vi "Get Write Mode.vi"(8 "error in (no error)":errorcluster, 11 "Item Ref in":T2 format="%.0x") -> (0 "error out":errorcluster, 2 "Write Mode":T1, 3 "Item Ref out":T2 format="%.0x")   [LabVIEW 2020, in "Modbus Master System Explorer.lvlib"]
uses:
  Modbus Master System Explorer.lvlib
  <vilib>/NI VeriStand/Custom Device API/Custom Device Item Ref.ctl
  Shared/Write Mode.ctl
  Shared/Constants.vi
  <vilib>/NI VeriStand/Custom Device API/Get Item Property (U16).vi
  Shared/Modbus Master Shared.lvlib
  <vilib>/NI VeriStand/Custom Device API/Custom Device API.lvlib
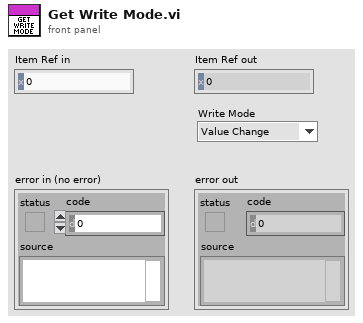
[diagram p1: front panel]
types:
  T1 = typedef "Modbus Master Shared.lvlib/Write Mode.ctl" = enum16{"Value Change", "Interval"}
  T2 = typedef "Custom Device API.lvlib/Custom Device Item Ref.ctl" = u64
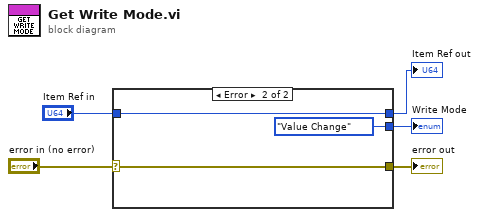
[diagram p0: block diagram]
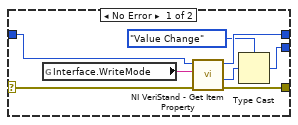
[diagram p2: hidden frame]
diagram:
  n1 = case shown="Error" "error in (no error)" {
    selector: "error in (no error)" -> [w12 w15]
    tunnel: "Item Ref in" -> [w11 w16]
    tunnel: [w10 w15] -> w3
    tunnel: [w9 w16] -> w2
    tunnel: [w6 Write_Mode."Value Change" ("Write Mode")] -> w1
    frame No Error {
      n2 = global read "Constants.vi" "Interface.WriteMode"() -> (w13:string)
      n3 = call-poly <vilib>:"NI VeriStand - Get Item Property.vi"("error in (no error)"=w12, "Property Name"=w13, "Item Ref in"=w11) -> ("error out"=w10:errorcluster, "Value"=w8:u16, "Item Ref out"=w9:T2)  [unwired: 5 in, 1 out]
      n4 = Type Cast(type=Write_Mode."Value Change" ("Write Mode"), x=w8) -> (*(type *) &x=w6:T1)
    }
    frame Error {
    }
  }
  "error out" <- w3
  "Item Ref out" <- w2
  "Write Mode" <- w1
